vi "Check For Messages.vi"(9 "Term Char":string="\r\n", 11 "Input String":string) -> (0 "found?":bool, 1 "data":u8[](array[numeric]), 3 "Remaining String":string)   [LabVIEW 2020, in "SubVIs.lvlib" / "ASCII Data Unit.lvclass"]
uses:
  <vilib>/Modbus/subvis/Transmission Data Unit (ADU)/ASCII Data Unit/ASCII Data Unit.lvclass
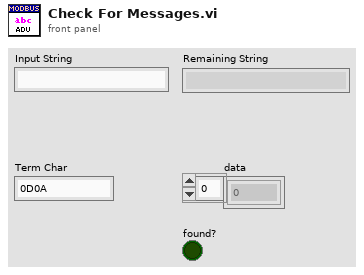
[diagram p1: front panel]
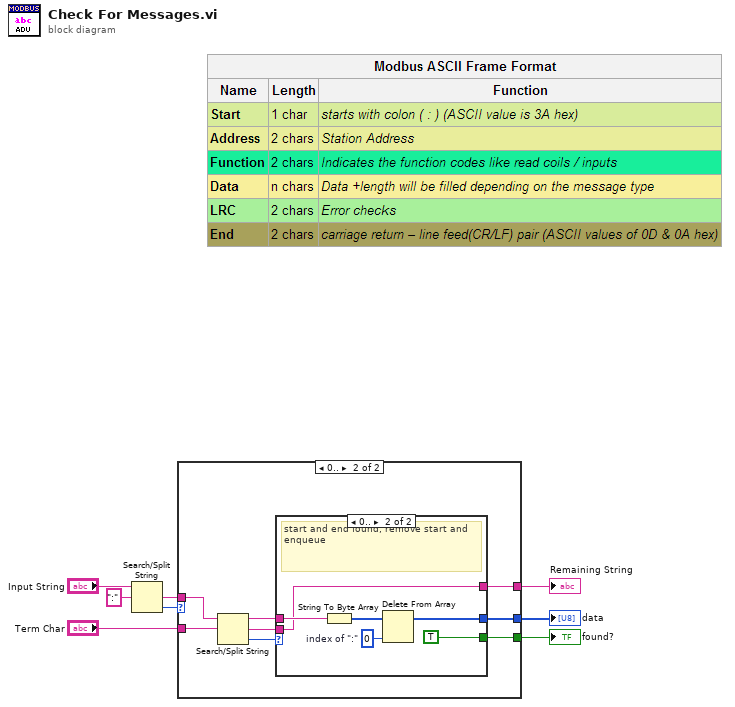
[diagram p0: block diagram]
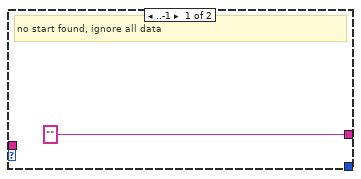
[diagram p2: hidden frame]
diagram:
  n1 = Search/Split String(string="Input String", search string/char (-)=":") -> (match + rest of string=w2:string, offset of match=w1:i32)  [unwired: 1 in, 1 out]
  n2 = case shown="0.." w1 {
    tunnel: "Term Char" -> [_ w17]
    tunnel: w2 -> [_ w16]
    tunnel: ["" ("Input String") w14] -> w6
    tunnel: [_ w11] -> w5
    tunnel: [_ w10] -> w4
    frame ..-1 {
      # "no start found, ignore all data"
    }
    frame 0.. {
      n3 = Search/Split String(string=w16, search string/char (-)=w17) -> (substring before match=w13:string, match + rest of string=w12:string, offset of match=w15:i32)  [unwired: 1 in]
      n4 = case shown="0.." w15 {
        tunnel: [w18 w21] -> w14
        tunnel: w13 -> [w18 w24]
        tunnel: w12 -> [_ w21]
        tunnel: [_ w20] -> w11
        tunnel: [_ TRUE] -> w10
        frame ..-1 {
          # "no term found yet, stop"
        }
        frame 0.. {
          w22 = 0  # index of ":"
          # "start and end found, remove start and enqueue"
          n5 = String To Byte Array(string=w24) -> (unsigned byte array=w23:u8[])
          n6 = Delete From Array(array=w23, index=w22) -> (array with subset deleted=w20:u8[])  [unwired: 1 in, 1 out]
        }
      }
    }
  }
  "Remaining String" <- w6
  "data" <- w5
  "found?" <- w4
